vi "Message.vi"() -> (0 "error out":errorcluster)   [LabVIEW 2017, in "Transparent Assertions.Tests.lvlib" / "Assert Count.lvlib"]
uses:
  Assert Count.lvlib
  src/Transparent Assertions/Transparent Assertions.lvlib
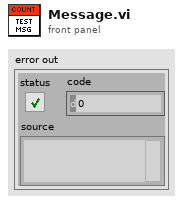
[diagram p1: front panel]
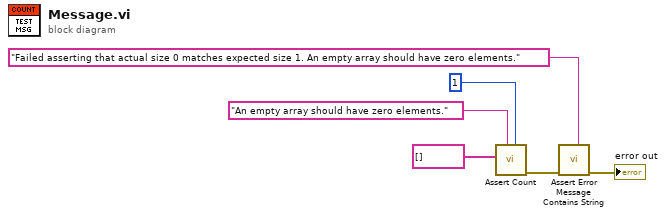
[diagram p0: block diagram]
diagram:
  n1 = call "Assert Count.vi"("Expected"=1, "Message (\"\")"="An empty array should have zero elements." ("Message (\"\")"), "Haystack"=string[] []) -> ("error out"=w6:errorcluster)  [unwired: 8 in]
  n2 = call "Assert Error Message Contains String.vi"("Expected"="Failed asserting that actual size 0 matches expected size 1. An empty array should have zero elements." ("y"), "error in (no error)"=w6) -> ("error out"=→"error out":errorcluster)  [unwired: 9 in]
